vi "_getDataPluginsExist.vi"(8 "error in (no error)":errorcluster, 11 "DataPlugin information in":T1[](array[typedef])) -> (0 "error out":errorcluster, 3 "DataPlugin information out":T1[](array[typedef]))   [LabVIEW 2017]
uses:
  <vilib>/Platform/storage/utility/DataPluginSynchronization/_DataPluginInfo.ctl
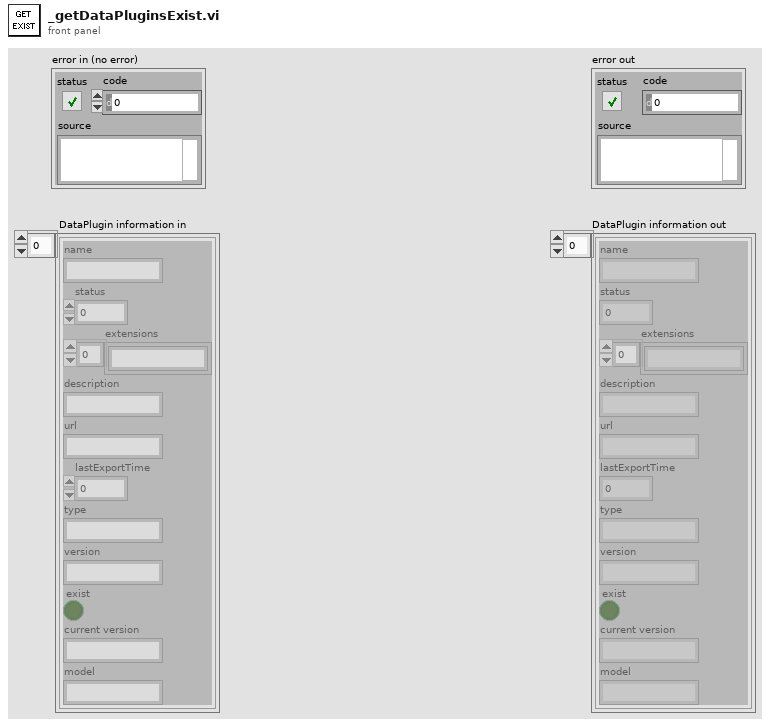
[diagram p1: front panel]
types:
  T1 = typedef "_DataPluginInfo.ctl" = cluster{"name":string, "status":u32, "extensions":string[], "description":string, "url":string, "lastExportTime":i64, "type":string, "version":string, "exist":bool, "current version":string, "model":string}
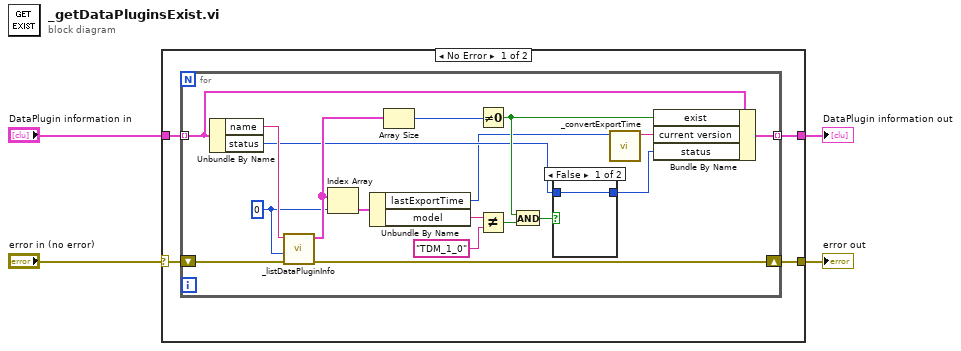
[diagram p0: block diagram]
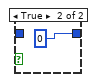
[diagram p2: hidden frame]
diagram:
  n1 = case shown="No Error" "error in (no error)" {
    selector: "error in (no error)" -> [w5 w29]
    tunnel: "DataPlugin information in" -> [w8 w30]
    tunnel: [w7 w30] -> w3
    tunnel: [w6 w29] -> w2
    frame No Error {
      n2 = for {
        tunnel: w8 -> [w26] mode=indexing
        tunnel: [w25] -> w7 mode=indexing
        shift-right: [w10] -> w6
        shift-left: w5 -> [w9]
        w11 = u32 0 ("source")
        n3 = Unbundle By Name(w26) -> ("name"=w23:string, "status"=w14:u32)
        n4 = call <vilib>:"_listDataPluginInfo.vi"("error in (no error)"=w9, "source"=w11, "DataPlugin name"=w23) -> ("error out"=w10:errorcluster, "DataPlugin information"=w22:T1[])  [unwired: 7 in]
        n5 = Index Array(array=w22, index=w11) -> (element=w24:T1)
        n6 = Unbundle By Name(w24) -> ("lastExportTime"=w13:i64, "model"=w20:string)
        n7 = Array Size(array=w22) -> (size(s)=w21:i32)
        n8 = Not Equal To 0?(x=w21) -> (x != 0?=w17:bool)
        n9 = Not Equal?(x=w20, y="TDM_1_0") -> (x != y?=w18:bool)
        n10 = And(x=w17, y=w18) -> (x .and. y?=w16:bool)
        n11 = case shown="False" w16 {
          tunnel: w14 -> [w27 _]
          tunnel: [w27 u32 0 ("status")] -> w15
          frame False {
          }
          frame True {
          }
        }
        n12 = call <vilib>:"_convertExportTime.vi"("lastExportTime"=w13) -> ("Time"=w12:string)  [unwired: 10 in]
        n13 = Bundle By Name(cluster=w26, "exist"=w17, "current version"=w12, "status"=w15) -> (w25:T1)
      }
    }
    frame Error {
    }
  }
  "DataPlugin information out" <- w3
  "error out" <- w2
